vi "Dashboard Main.vi"() -> ()   [LabVIEW 2017]
uses:
  <vilib>/event_ctls.llb/eventvkey.ctl
  <vilib>/Rock Robotics/WPI/Dashboard/WPI_DashboardLogging Global.vi
  <vilib>/Utility/miscctls.llb/LVRowAndColumnTypeDef.ctl
  <vilib>/Rock Robotics/Network Tables/NT Write Boolean.vi
  <vilib>/Rock Robotics/Network Tables/NT Read Numeric Array.vi
panel:
  out "error out":errorcluster
  out "error out 2":errorcluster
  in  "Camera Settings Right":T1={"Frame Rate"=30, "Compression"=30, "Size"=1, "DB Camera Config"=FALSE} {"Frame Rate" scale=1.0..30.0; "Compression" scale=100.0..-1.0; "Size" items=["640x480", "320x240", "160x120"]}
  in  "Camera Name Right":string(combo)="No Camera Selection"
  out "Camera Info":cluster{"Mbps LED":bool, "Mbps":dbl, "fps":dbl} {"fps" format="%#.1g"; "Mbps" format="%#.1g"}
  in  "Camera Settings":T1={"Frame Rate"=30, "Compression"=30, "Size"=1, "DB Camera Config"=FALSE} {"Frame Rate" scale=1.0..30.0; "Compression" scale=100.0..-1.0; "Size" items=["640x480", "320x240", "160x120"]}
  in  "TCP":refnum<k5>
  in  "Rec Mode":enum32{"Stop", "Record", "Playback"}(radio)
  out "Robot IP":string
  out "Image Message":string="Timeout in Camera Communications"
  in  "Dashboard Tab":T2(tab)
  in  "Select Auto":string(combo)="Select Autonomous ..."
  out "NT Connection":bool
  out "MotorChart R":cluster{"Numeric":dbl, "Numeric":dbl}(graph)
  out "MotorChart L":cluster{"Numeric":dbl, "Numeric":dbl}(graph)
  out "MotorSliders R":cluster{"MotorSlide1":dbl, "MotorSlide2":dbl} {"MotorSlide2" scale=-1.0..1.0 scale format="%#_2e"; "MotorSlide1" scale=-1.0..1.0 scale format="%#_2e"}
  out "MotorSliders L":cluster{"MotorSlide1":dbl, "MotorSlide2":dbl} {"MotorSlide2" scale=-1.0..1.0 scale format="%#_2e"; "MotorSlide1" scale=-1.0..1.0 scale format="%#_2e"}
  out "JS1 Z":dbl(slide) scale=-1.0..1.0 scale format="%#_2e"
  out "JS1 Graph":cluster{"X":dbl, "Y":dbl}[](graph)
  out "JS1 Buttons":T3
  out "JS2 Z":dbl(slide) scale=-1.0..1.0 scale format="%#_2e"
  out "JS2 Graph":cluster{"X":dbl, "Y":dbl}[](graph)
  out "JS2 Buttons":T3
  out "Mode":T4(ring)=enum."Auto Disabled"
  out "Gear State":string="Waiting...."
  in  "Mode 2":bool
  out "Camera Image Right":T5(plugin-control)
  in  "DB/String 9":string
  in  "DB/String 8":string
  in  "DB/String 7":string
  in  "DB/String 6":string
  in  "DB/String 5":string
  in  "DB/String 4":string
  in  "DB/String 3":string
  in  "DB/String 2":string
  in  "DB/String 1":string
  in  "DB/String 0":string
  in  "DB/Slider 0":dbl(slide) scale=0.0..5.0
  in  "DB/Slider 1":dbl(slide) scale=0.0..5.0
  in  "DB/Slider 2":dbl(slide) scale=0.0..5.0
  in  "DB/Slider 3":dbl(slide) scale=0.0..5.0
  out "DB/LED 3":bool
  out "DB/LED 2":bool
  out "DB/LED 1":bool
  out "DB/LED 0":bool
  in  "DB/Button 3":bool
  in  "DB/Button 2":bool
  in  "DB/Button 1":bool
  in  "DB/Button 0":bool caption="New Name"
  in  "Test Slider":dbl(slide) scale=0.0..100.0 scale format="%#_3g"
  in  "On/Off":bool caption="Solenoid"
  in  "Test Name":u16(ring) items=["Select the test to run..."]
  in  "Test Tree":string(tree)
  in  "Motor":cluster{"Value":dbl, "Enable":bool} {"Value" scale=-1.0..1.0 scale format="%#_3g"}
  out "Progress":T6 {"Test Progress" scale=0.0..100.0}
  in  "Rev/Fwd":cluster{"Forward":bool, "Reverse":bool}
  in  "Test Ring":u16(ring) items=["Monochrome", "Color"]
  out "Cmd Status":string
  in  "Execute Command":bool
  in  "Command Params":string[][](table)
  in  "Command Selection":i32(listbox)
  in  "CheckList":i32(listbox)
  out "Tree":string(tree)
  in  "Max Speed":dbl=1.0 format="%#_13g"
  in  "Foreward Sensitivity":dbl=1.0 format="%#_13g"
  in  "Turning Sensitivity":dbl=0.4 format="%#_13g"
  in  "High Gear Turning Multiplier":dbl=0.65 format="%#_13g"
  in  "High Gear":bool=TRUE
  in  "Direction Toggle":bool=TRUE
  in  "Autoshift":bool=TRUE
  in  "Save":bool
  in  "Load":bool
  in  "Profile Name":string="Profile1"
  out "Camera Image":T5(plugin-control)
  out "Background":bool
  in  "Camera Name":string(combo)="No Camera Selection"
  # "HW"
  # "HW"
  # "Joysticks"
  # "Drive Motors"
  # "Front"
  # "Right"
  # "Left"
  # "Back"
  # "This tab is a great place for autonomous settings and robot-specific values.\nPlace controls and indicators inside this tab and match name to\nDashboard Variables on robot. You can also delete this comment."
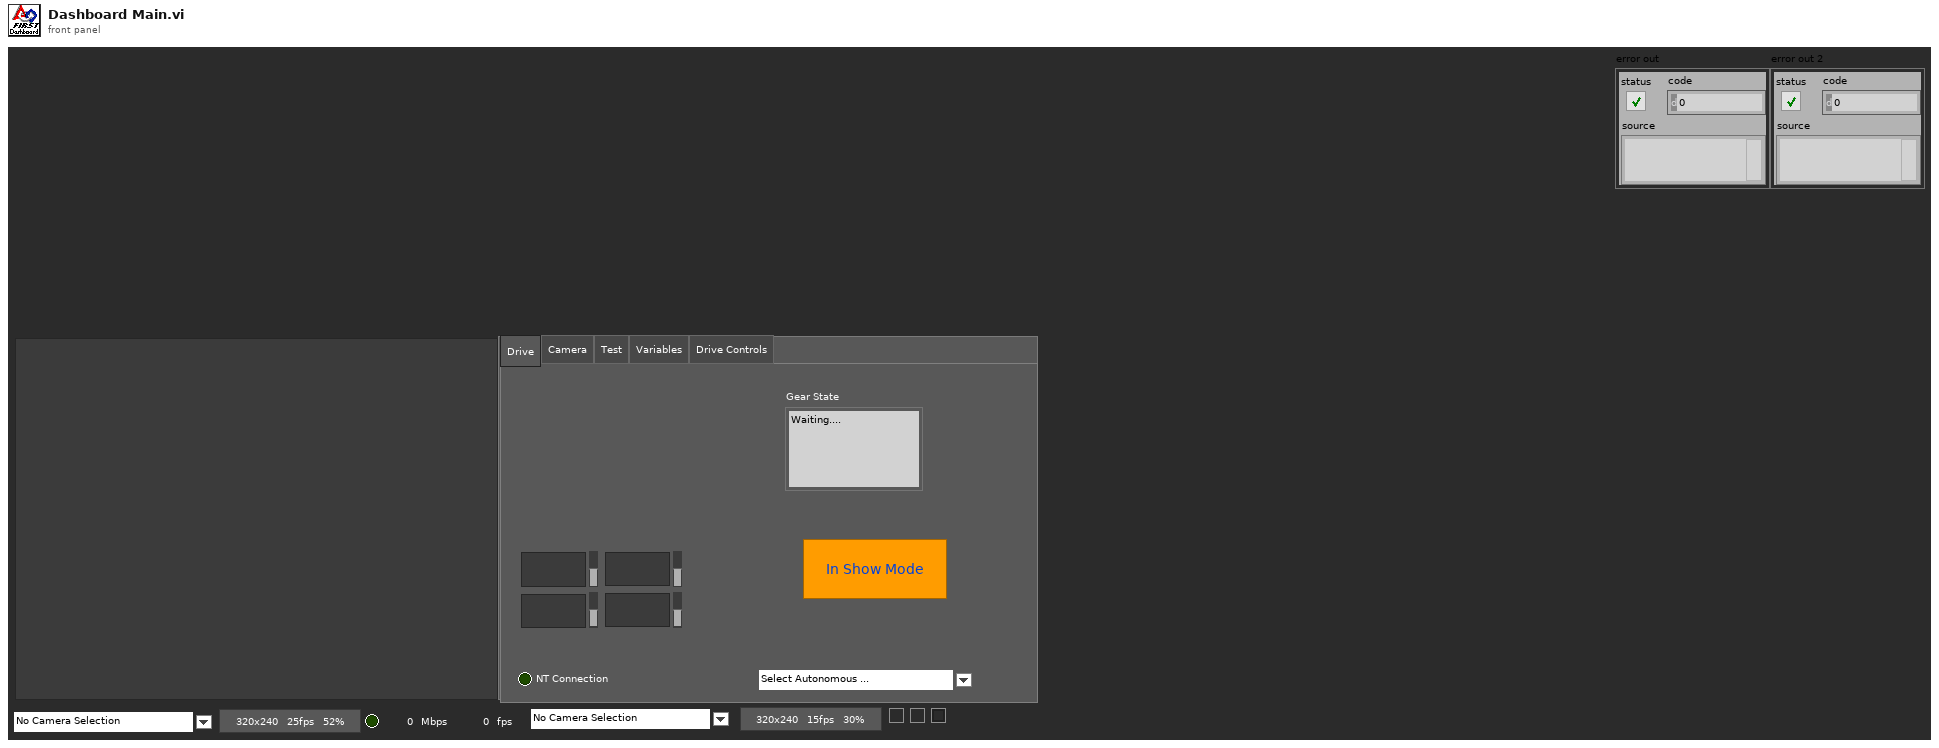
[diagram p1: front panel]
types:
  T1 = cluster{"Frame Rate":i32, "Compression":i32, "Size":u16, "DB Camera Config":bool}
  T2 = enum32{"Drive", "Camera", "Basic", "Custom", "Test", "Commands", "Checklist", "Variables", "Drive Controls"}
  T3 = cluster{bool, bool, bool, bool, bool, bool, bool, bool, bool, bool, bool, bool}
  T4 = enum8{"Tele-Op Disabled", "Tele-Op Enabled", "Auto Disabled", "Auto Enabled", "Test Disabled", "Test Enabled", "Disconnected", "No Code", "E-Stop"}
  T5 = typedef "IMAQ Image.ctl" = refnum<image>
  T6 = cluster{"Test Progress":u8, "Test Progress Text":string}
  T7 = typedef "Image Type" = u32
  T8 = cluster{"IDs":cluster{"RPC field ID":u16, "Unique ID":u16}, "String":string}
  T9 = enum32{"Drive", "Camera", "Basic", "Custom", "Test", "Commands", "Checklist", "Variables"}
  T10 = enum32{"Drive", "Basic", "Custom", "Test", "Checklist", "Variables"}
  T11 = cluster{"Error Strings":string, "Disable Counts":cluster{u16, u16}, "Rail Faults":cluster{u16, u16, u16}, "Robot IP":string, "DB Mode":u8, "Event Info":cluster{"Name":string, "Type":u8, "Number":u16, "Replay":u8}}
  T12 = cluster{"Storage":cluster{"Disk Free":u64, "RAM Block":u32, "RAM free":u32}, "CPU Utilization":cluster{"CPU % ISR":sgl, "CPU % Time Crit":sgl, "CPU % Timed Str":sgl, "CPU % High":sgl, "CPU % Above":sgl, "CPU % Normal":sgl, "CPU % Low":sgl}, "CAN":cluster{"% Bus Utilization":sgl, "Bus Off Cnt":u32, "TX_FIFO Full Cnt":u32, "Receive Error Cnt":u8, "Transmit Error Cnt":u8}, "HID":cluster{"HID Outputs":u32, "Rumble Low":u16, "Rumble High":u16}[]}
  T13 = cluster{"Status bits":cluster{"Test Mode":bool, "Autonomous":bool, "Enabled":bool, "Code Start":bool, "Brownout":bool, "Reserved 2":bool, "Reserved 3":bool, "E-Stop":bool}, "Code Trace":cluster{"Disabled":bool, "TeleOp":bool, "Auto":bool, "Test":bool}, "Controller Type":enum16{"unknown", "cRIO", "roboRio"}, "Code?":enum16{"unknown", "noCode", "code"}, "Battery V":dbl}
  T14 = cluster{"Control Bits":cluster{"TestMode":bool, "Autonomous":bool, "Enabled":bool, "FMS Present":bool, bool, bool, bool, "E-Stop":bool}, "Team Station ":u8, "Countdown":sgl, "Joystick Values":cluster{"Axes":dbl[], "Buttons":bool[], "POVs":i16[]}[]}
  T15 = cluster{"Axes":dbl[], "Buttons":bool[], "POVs":i16[]}[]
  T16 = cluster{"Axes":dbl[], "Buttons":bool[], "POVs":i16[]}
  T17 = cluster{"Buttons[0]":bool, "Buttons[1]":bool, "Buttons[2]":bool, "Buttons[3]":bool, "Buttons[4]":bool, "Buttons[5]":bool, "Buttons[6]":bool, "Buttons[7]":bool, "Buttons[8]":bool, "Buttons[9]":bool, "Buttons[10]":bool, "Buttons[11]":bool}
  T18 = cluster{"High Gear Turning Multiplier":refnum<vi>, "Turning Sensitivity":refnum<vi>, "Foreward Sensitivity":refnum<vi>, "Max Speed":refnum<vi>, "Autoshift":refnum<vi>, "High Gear":refnum<vi>, "Direction Toggle":refnum<vi>, "Profile Name":refnum<vi>}
  T19 = cluster{"Camera Image":refnum<vi>, "Dashboard Tab":refnum<vi>, "Background":refnum<vi>, "Rec Mode":refnum<vi>, "Test Slider":refnum<vi>, "On/Off ":refnum<vi>, "Test Ring":refnum<vi>, "Rev/Fwd":refnum<vi>, "Test Name":refnum<vi>, "Motor":refnum<vi>, "Progress":refnum<vi>, "CheckList":refnum<vi>, "Tree":refnum<vi>, "Test Tree":refnum<vi>, "Command Params":refnum<vi>, "Command Selection":refnum<vi>, "Execute Command":refnum<vi>, "Cmd Status":refnum<vi>, "Camera Settings":refnum<vi>, "Camera Name":refnum<vi>, "Camera Info":refnum<vi>, "Camera Settings Right":refnum<vi>, "Camera Name Right":refnum<vi>, "Camera Image Right":refnum<vi>}
  T20 = cluster{"Operation":enum16{"Update", "Clear"}, "Color Box":u32}[]
  T21 = typedef "eventvkey.ctl" = enum16{"ASCII", "Enter", "Return", "Shift", "Ctrl", "Alt", "Cmd", "Opt", "Caps", "NumLock", "Clear", "Break", "Up", "Down", "Left", "Right", "Insert", "Delete", "Home", "End", "PageUp", "PageDown", "Escape", "Help", "Pause", "ScrollLock", "F1", "F2", "F3", "F4", "F5", "F6", "F7", "F8", "F9", "F10", "F11", "F12", "F13", "F14", "F15", "F16", "F17", "F18", "F19", "F20", "F21", "F22", "F23", "F24", "Play", "VolumeUp", "VolumeDown", "Mute", "Two Byte Char"}
  T22 = cluster{"Image Size":bool, "Image Type":bool, "Pixel Value":bool, "ROI Information":bool, "Zoom Factor":bool}
  T23 = cluster{"Operation":enum16{"Update", "Clear"}, "Color Box":u32}
  T24 = typedef "LVRowAndColumnTypeDef.ctl" = cluster{"Row":i32, "Column":i32}
  T25 = cluster{"Shift":bool, "Ctrl":bool, "Alt":bool, "Cmd":bool, "Opt":bool}
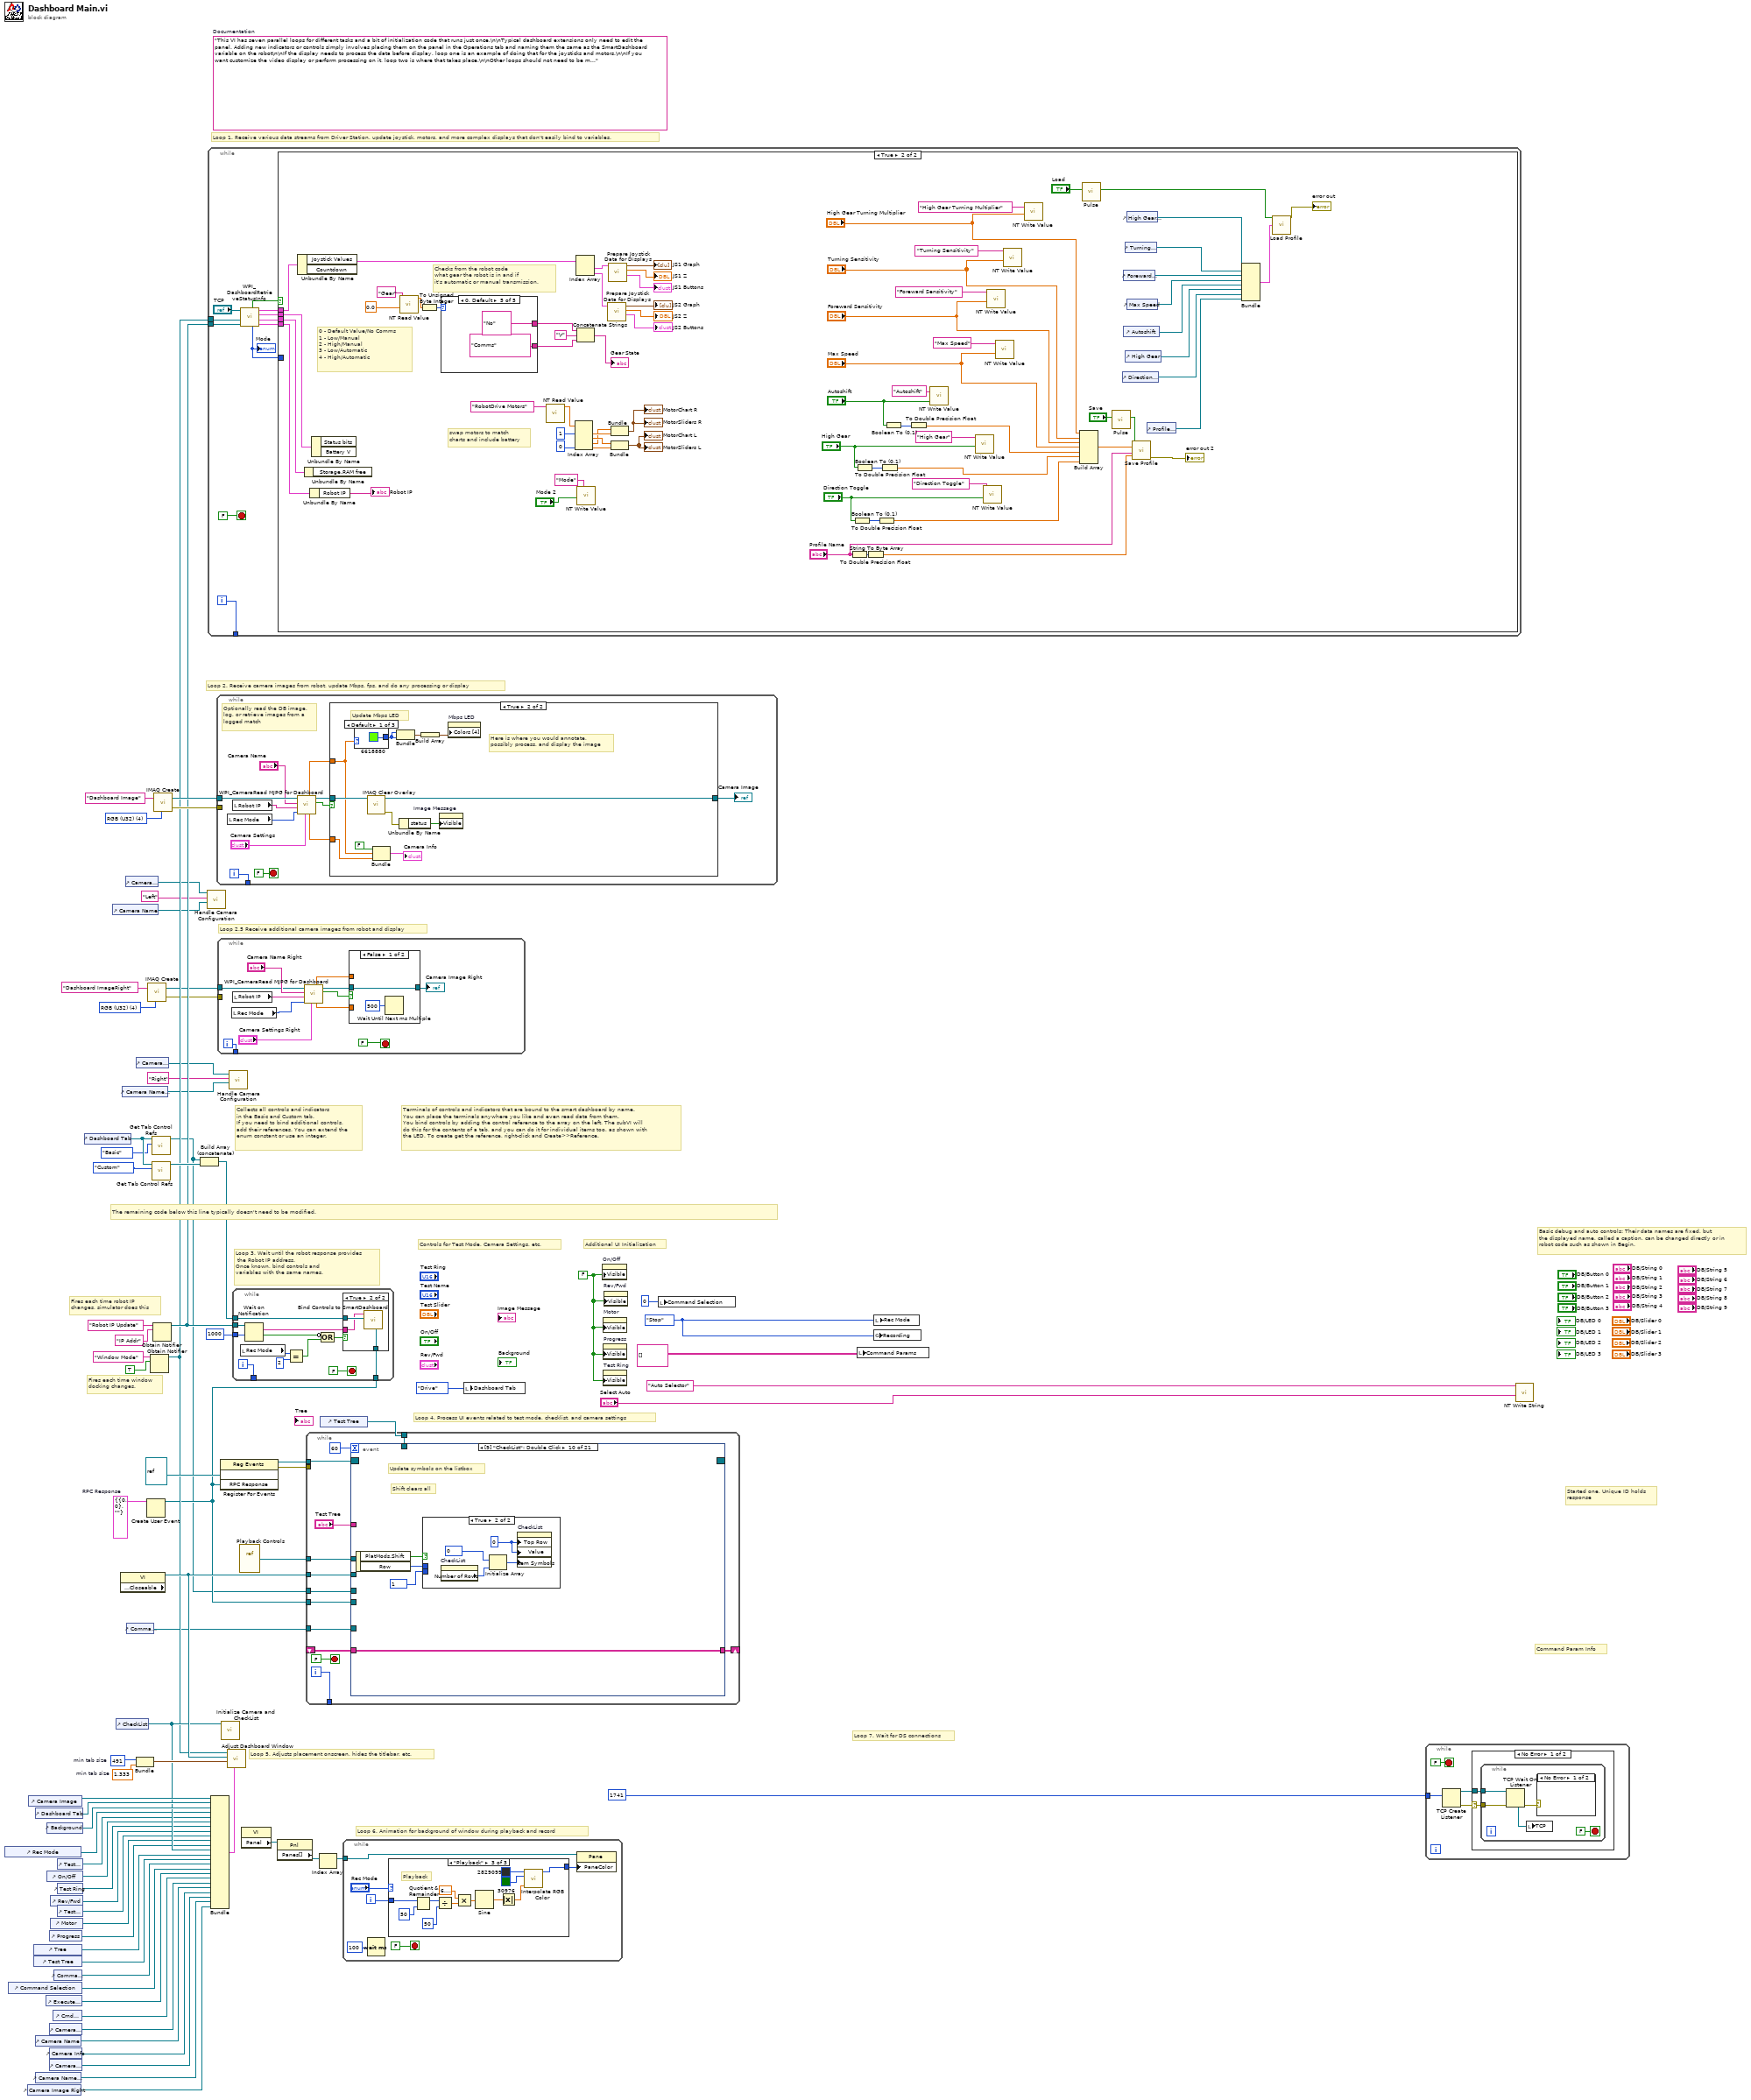
[diagram p0: block diagram]
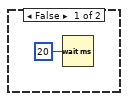
[diagram p3: hidden frame]
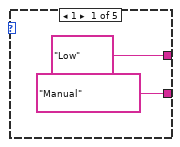
[diagram p4: hidden frame]
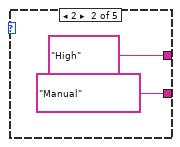
[diagram p5: hidden frame]
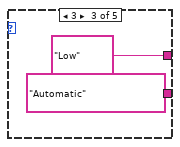
[diagram p6: hidden frame]
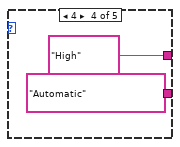
[diagram p7: hidden frame]
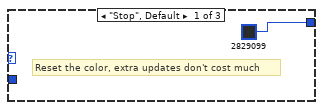
[diagram p8: hidden frame]
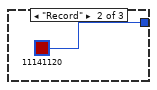
[diagram p9: hidden frame]
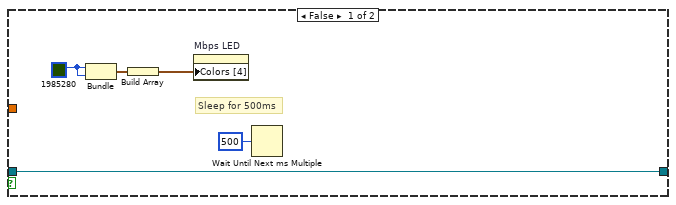
[diagram p11: hidden frame]
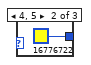
[diagram p12: hidden frame]
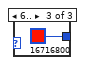
[diagram p13: hidden frame]
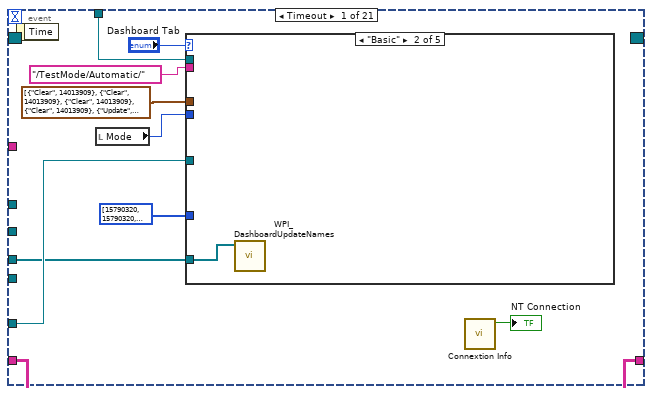
[diagram p14: hidden frame]
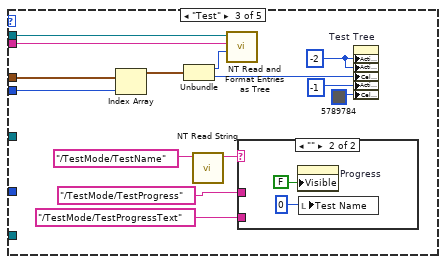
[diagram p16: hidden frame]
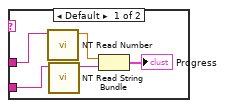
[diagram p17: hidden frame]
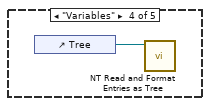
[diagram p18: hidden frame]
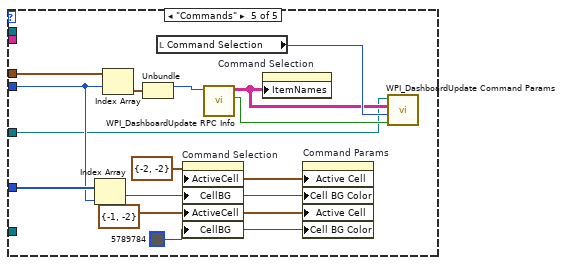
[diagram p19: hidden frame]
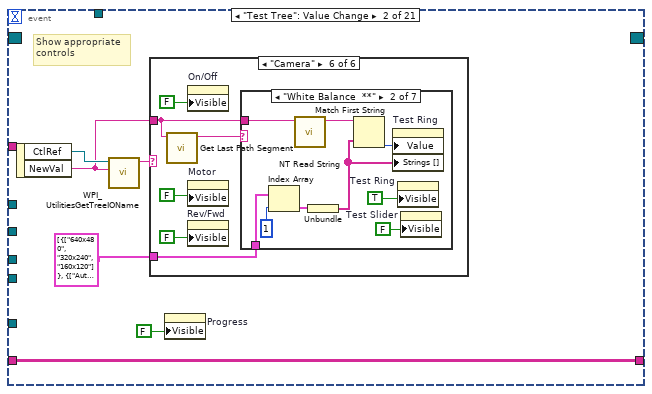
[diagram p20: hidden frame]
diagram:
  w10 = T7 4 items=["Grayscale (U8)", "Grayscale (I16)", "Grayscale (SGL)", "Complex (CSG)", "RGB (U32)", "HSL (U32)", "RGB (U64)"] ("Image Type")
  w26 = T8 {"IDs"={"RPC field ID"=0, "Unique ID"=0}, "String"=""}  # RPC Response
  w51 = 491  # min tab size
  w50 = 1.333  # min tab size
  w58 = enum32{"Stop", "Record", "Playback"}."Stop" ("Rec Mode")
  w33 = FALSE ("Visible")
  (unwired) "This VI has seven parallel loops for different tasks and a bit of initialization code that runs just once.\n\nTypical dashboard extensions only need to edit the panel. Adding new indicators or controls simply involves placing them on the panel in the Operations tab and naming them the same as the SmartDashboard variable on the robot\n\nIf the display needs to process the data before display, loop one is an example of doing that for the joysticks and motors.\n\nIf you want customize the video display or perform processing on it, loop two is where that takes place.\n\nOther loops should not need to be modified. They are pretty standard, and document the task they perform."  # Documentation
  w75 = T7 4 items=["Grayscale (U8)", "Grayscale (I16)", "Grayscale (SGL)", "Complex (CSG)", "RGB (U32)", "HSL (U32)", "RGB (U64)"] ("Image Type")
  # "Loop 2.5 Receive additional camera images from robot and display"
  # "Command Param Info"
  # "Started one, Unique ID holds\nresponse"
  # "Loop 7. Wait for DS connections"
  # "Basic debug and auto controls: Their data names are fixed, but\nthe displayed name, called a caption, can be changed directly or in\nrobot code such as shown in Begin."
  # "Controls for Test Mode, Camera Settings, etc."
  # "Additional UI Initialization"
  # "Loop 6. Animation for background of window during playback and record"
  # "Fires each time robot IP\nchanges, simulator does this"
  # "Fires each time window\ndocking changes."
  # "Collects all controls and indicators\nin the Basic and Custom tab.\nIf you need to bind additional controls,\nadd their references. You can extend the\nenum constant or use an integer."
  # "The remaining code below this line typically doesn't need to be modified."
  # "Loop 4. Process UI events related to test mode, checklist, and camera settings"
  # "Terminals of controls and indicators that are bound to the smart dashboard by name.\nYou can place the terminals anywhere you like and even read data from them.\nYou bind controls by adding the control reference to the array on the left. The subVI will\ndo this for the contents of a tab, and you can do it for individual items too, as shown with\nthe LED. To create get the reference, right-click and Create>>Reference."
  # "Loop 3. Wait until the robot response provides\n the Robot IP address.\nOnce known, bind controls and\nvariables with the same names."
  # "Loop 5. Adjusts placement onscreen, hides the titlebar, etc."
  # "Loop 1. Receive various data streams from Driver Station, update joystick, motors, and more complex displays that don't easily bind to variables."
  # "Loop 2. Receive camera images from robot, update Mbps, fps, and do any processing or display"
  n1 = control-ref of="Rec Mode"() -> (w39:refnum<vi>)
  n2 = control-ref of="Command Selection"() -> (w25:refnum<vi>)
  n3 = control-ref of="Camera Image Right"() -> (w1:refnum<vi>)
  n4 = control-ref of="Camera Image"() -> (w53:refnum<vi>)
  n5 = control-ref of="Tree"() -> (w43:refnum<vi>)
  n6 = control-ref of="Test Tree"() -> (w42:refnum<vi>)
  n7 = control-ref of="Dashboard Tab"() -> (w52:refnum<vi>)
  n8 = control-ref of="Camera Name"() -> (w16:refnum<vi>)
  n9 = control-ref of="Camera Name Right"() -> (w2:refnum<vi>)
  n10 = control-ref of="Execute Command"() -> (w27:refnum<vi>)
  n11 = control-ref of="Background"() -> (w48:refnum<vi>)
  n12 = control-ref of="On/Off"() -> (w37:refnum<vi>)
  n13 = control-ref of="Progress"() -> (w34:refnum<vi>)
  n14 = control-ref of="Camera Settings"() -> (w17:refnum<vi>)
  n15 = control-ref of="Camera Info"() -> (w15:refnum<vi>)
  n16 = control-ref of="Camera Settings Right"() -> (w3:refnum<vi>)
  n17 = control-ref of="Rev/Fwd"() -> (w35:refnum<vi>)
  n18 = control-ref of="Motor"() -> (w40:refnum<vi>)
  n19 = control-ref of="Cmd Status"() -> (w21:refnum<vi>)
  n20 = control-ref of="Command Params"() -> (w28:refnum<vi>)
  n21 = control-ref of="Test Slider"() -> (w38:refnum<vi>)
  n22 = control-ref of="Test Ring"() -> (w36:refnum<vi>)
  n23 = control-ref of="Test Name"() -> (w41:refnum<vi>)
  n24 = control-ref of="Dashboard Tab"() -> (w56:refnum<vi>)
  n25 = control-ref of="Camera Name"() -> (w18:refnum<vi>)
  n26 = control-ref of="CheckList"() -> (w44:refnum<vi>)
  n27 = property class="VI" props=["Front Panel.Closeable"]() -> (reference out=w57:refnum<vi>)  [unwired: 2 in, 2 out]
  n28 = control-ref of="Camera Name Right"() -> (w6:refnum<vi>)
  n29 = control-ref of="Camera Settings"() -> (w19:refnum<vi>)
  n30 = control-ref of="Command Params"() -> (w20:refnum<vi>)
  n31 = control-ref of="Camera Settings Right"() -> (w7:refnum<vi>)
  n32 = Bundle("min tab size"=w51, "min tab size"=w50) -> (w49:cluster{"min tab size":i32, "min tab size":dbl})  [unwired: 1 in]
  n33 = Create User Event(user event datatype=w26) -> (user event=w22:refnum<user-event>)  [unwired: 1 in, 1 out]
  n34 = call "IMAQ Create"("Image Name"="Dashboard ImageRight", "Image Type"=w10) -> ("New Image"=w9:T5, "error out"=w8:errorcluster)  [unwired: 2 in, 1 out]
  n35 = Obtain Notifier(name (unnamed)="Window Mode", notification data type=TRUE) -> (notifier out=w31:refnum<notifier>)  [unwired: 2 in, 2 out]
  n36 = call <vilib>:"Get Tab Control Refs.vi"("Page Index"=T10."Basic" ("Dashboard Tab"), "TabControl in"=w56) -> ("ControlsOnPage"=w14:refnum<vi>[])  [unwired: 9 in]
  n37 = call <vilib>:"Get Tab Control Refs.vi"("Page Index"=T10."Custom" ("Dashboard Tab"), "TabControl in"=w56) -> ("ControlsOnPage"=w55:refnum<vi>[])  [unwired: 9 in]
  n38 = Obtain Notifier(name (unnamed)="Robot IP Update", notification data type="IP Addr" ("name (unnamed)")) -> (notifier out=w32:refnum<notifier>)  [unwired: 2 in, 2 out]
  n39 = call "IMAQ Create"("Image Name"="Dashboard Image", "Image Type"=w75) -> ("New Image"=w73:T5, "error out"=w72:errorcluster)  [unwired: 2 in, 1 out]
  n40 = Build Array (concatenate)(w14, w55) -> (w54:refnum<vi>[])
  n41 = call "Handle Camera Configuration.vi"("CameraNameRef"=w18, "Camera File Name"="Left", "ClusterRef"=w19) -> ()  [unwired: 9 in]
  n42 = while {
    tunnel: [w85] -> _
    tunnel: w32 -> [w79]
    tunnel: w31 -> [w76]
    i -> [w85]
    stop <- FALSE stop-if-true
    n43 = call <vilib>:"WPI_DashboardRetrieveStatusInfo.vi"("Binding Refnum"=w79, "Window Mode Notifier"=w76, "TCP Cnx"="TCP") -> ("Power and Errors"=w80:T11, "Robot Metrics"=w83:T12, "Status Info"=w84:T13, "Control Info"=w81:T14, "Robot Mode"=w78:T4, "Process?"=w82:bool)  [unwired: 3 in]
    "Mode" <- w78
    n44 = case shown="True" w82 {
      tunnel: w84 -> [_ w160]
      tunnel: w83 -> [_ w159]
      tunnel: w81 -> [_ w158]
      tunnel: w80 -> [_ w157]
      tunnel: w78 -> [_ _]
      frame False {
        n45 = Wait (ms)(milliseconds to wait=u32 20) -> ()  [unwired: 1 out]
      }
      frame True {
        # "Checks from the robot code\nwhat gear the robot is in and if\nit's automatic or manual transmission."
        # "0 - Default Value/No Comms\n1 - Low/Manual\n2 - High/Manual\n3 - Low/Automatic\n4 - High/Automatic"
        # "swap motors to match\ncharts and include battery"
        n46 = Unbundle By Name(w158) -> ("Joystick Values"=w148:T15)  [unwired: 1 out]
        n47 = Unbundle By Name(w159) -> ()  [unwired: 1 out]
        n48 = Unbundle By Name(w157) -> ("Robot IP"=→"Robot IP":string)
        n49 = Unbundle By Name(w160) -> ()  [unwired: 2 out]
        n50 = call-poly <vilib>:"NT Read Value.vi"("Default Value"=0.0, "Name"="Gear") -> ("Numeric"=w129:dbl)  [unwired: 8 in, 1 out]
        n51 = To Unsigned Byte Integer(number=w129) -> (unsigned 8bit integer=w130:u8)
        n52 = case shown="0, Default" w130 {
          tunnel: ["Low" "High" "Low" "High" "No"] -> w134
          tunnel: ["Manual" "Manual" "Automatic" "Automatic" "Comms"] -> w132
          frame 1 {
          }
          frame 2 {
          }
          frame 3 {
          }
          frame 4 {
          }
          frame 0, Default {
          }
        }
        n53 = call-poly <vilib>:"NT Read Value.vi"("Name"="RobotDrive Motors") -> ("Numeric Array"=w138:dbl[])  [unwired: 9 in, 1 out]
        n54 = Index Array(array=w138, index #1=1, index #4=0) -> (element #1=w152:dbl, element #2=w153:dbl, element #3=w151:dbl, element #4=w156:dbl)  [unwired: 2 in]
        n55 = Index Array(array=w148) -> (element #1=w147:T16, element #2=w143:T16)  [unwired: 2 in]
        n56 = Concatenate Strings(w134, "\r", w132) -> (→"Gear State":string)
        n57 = call-poly <vilib>:"NT Write Value.vi"("Boolean"="Mode 2", "Name"="Mode") -> ()  [unwired: 9 in, 1 out]
        n58 = call "Prepare Joystick Data for Displays.vi"("Joystick Values"=w143) -> ("Buttons"=→"JS2 Buttons":T17, "Z Axis"=→"JS2 Z":dbl, "Cartesian Data"=→"JS2 Graph":cluster{"X axis":dbl, "X axis":dbl}[])  [unwired: 8 in]
        n59 = call "Prepare Joystick Data for Displays.vi"("Joystick Values"=w147) -> ("Buttons"=→"JS1 Buttons":T17, "Z Axis"=→"JS1 Z":dbl, "Cartesian Data"=→"JS1 Graph":cluster{"X axis":dbl, "X axis":dbl}[])  [unwired: 8 in]
        n60 = Bundle("Numeric"=w151, "Numeric"=w152) -> (→"MotorChart R" →"MotorSliders R":cluster{"Numeric":dbl, "Numeric":dbl})  [unwired: 1 in]
        n61 = Bundle("Numeric"=w153, "Numeric"=w156) -> (→"MotorChart L" →"MotorSliders L":cluster{"Numeric":dbl, "Numeric":dbl})  [unwired: 1 in]
        n62 = String To Byte Array(string="Profile Name") -> (unsigned byte array=w109:u8[])
        n63 = Boolean To (0,1)(Boolean="Direction Toggle") -> (0, 1=w106:i16)
        n64 = Boolean To (0,1)(Boolean="High Gear") -> (0, 1=w104:i16)
        n65 = To Double Precision Float(number=w109) -> (double precision float=w111:dbl[])
        n66 = To Double Precision Float(number=w106) -> (double precision float=w107:dbl)
        n67 = To Double Precision Float(number=w104) -> (double precision float=w105:dbl)
        n68 = Boolean To (0,1)(Boolean="Autoshift") -> (0, 1=w102:i16)
        n69 = To Double Precision Float(number=w102) -> (double precision float=w103:dbl)
        n70 = call-poly <vilib>:"NT Write Value.vi"("Boolean"="Autoshift", "Name"="Autoshift") -> ()  [unwired: 9 in, 1 out]
        n71 = call-poly <vilib>:"NT Write Value.vi"("Boolean"="High Gear", "Name"="High Gear") -> ()  [unwired: 9 in, 1 out]
        n72 = call-poly <vilib>:"NT Write Value.vi"("Boolean"="Direction Toggle", "Name"="Direction Toggle") -> ()  [unwired: 9 in, 1 out]
        n73 = call-poly <vilib>:"NT Write Value.vi"("Numeric"="Foreward Sensitivity", "Name"="Foreward Sensitivity") -> ()  [unwired: 9 in, 1 out]
        n74 = call-poly <vilib>:"NT Write Value.vi"("Numeric"="Max Speed", "Name"="Max Speed") -> ()  [unwired: 9 in, 1 out]
        n75 = call-poly <vilib>:"NT Write Value.vi"("Numeric"="Turning Sensitivity", "Name"="Turning Sensitivity") -> ()  [unwired: 9 in, 1 out]
        n76 = call-poly <vilib>:"NT Write Value.vi"("Numeric"="High Gear Turning Multiplier", "Name"="High Gear Turning Multiplier") -> ()  [unwired: 9 in, 1 out]
        n77 = Build Array("High Gear Turning Multiplier", "Turning Sensitivity", "Foreward Sensitivity", "Max Speed", w103, w105, w107) -> (w110:dbl[])
        n78 = call "Pulse.vi"("Input"="Load") -> ("Output"=w98:bool)  [unwired: 10 in]
        n79 = call "Pulse.vi"("Input"="Save") -> ("Output"=w101:bool)  [unwired: 10 in]
        n80 = control-ref of="Direction Toggle"() -> (w90:refnum<vi>)
        n81 = control-ref of="Autoshift"() -> (w92:refnum<vi>)
        n82 = control-ref of="Foreward Sensitivity"() -> (w94:refnum<vi>)
        n83 = control-ref of="High Gear"() -> (w91:refnum<vi>)
        n84 = control-ref of="Turning Sensitivity"() -> (w95:refnum<vi>)
        n85 = control-ref of="High Gear Turning Multiplier"() -> (w96:refnum<vi>)
        n86 = control-ref of="Max Speed"() -> (w93:refnum<vi>)
        n87 = call "Save Profile.vi"("Array 2"=w111, "Profile Name"="Profile Name", "Array"=w110, "Output"=w101) -> ("error out"=→"error out 2":errorcluster)  [unwired: 7 in]
        n88 = control-ref of="Profile Name"() -> (w89:refnum<vi>)
        n89 = Bundle("High Gear Turning Multiplier"=w96, "Turning Sensitivity"=w95, "Foreward Sensitivity"=w94, "Max Speed"=w93, "Autoshift"=w92, "High Gear"=w91, "Direction Toggle"=w90, "Profile Name"=w89) -> (w88:T18)  [unwired: 1 in]
        n90 = call "Load Profile.vi"("Output"=w98, "output cluster"=w88) -> ("error out"=→"error out":errorcluster)  [unwired: 13 in]
      }
    }
  }
  n91 = Bundle("Camera Image"=w53, "Dashboard Tab"=w52, "Background"=w48, "Rec Mode"=w39, "Test Slider"=w38, "On/Off"=w37, "Test Ring"=w36, "Rev/Fwd"=w35, "Test Name"=w41, "Motor"=w40, "Progress"=w34, "CheckList"=w44, "Tree"=w43, "Test Tree"=w42, "Command Params"=w28, "Command Selection"=w25, "Execute Command"=w27, "Cmd Status"=w21, "Camera Settings"=w17, "Camera Name"=w16, "Camera Info"=w15, "Camera Settings Right"=w3, "Camera Name Right"=w2, "Camera Image Right"=w1) -> (w45:T19)  [unwired: 1 in]
  n92 = while {
    tunnel: w73 -> [w180]
    tunnel: w72 -> [_]
    tunnel: [w181] -> _
    i -> [w181]
    stop <- FALSE stop-if-true
    # "Optionally read the DB image,\nlog, or retrieve images from a\nlogged match"
    n93 = local read "Rec Mode"() -> (w176:enum32{"Stop", "Record", "Playback"})
    n94 = local read "Robot IP"() -> (w175:string)
    n95 = call <vilib>:"WPI_CameraRead MJPG for Dashboard.vi"("Camera Settings"="Camera Settings", "Rec Mode"=w176, "NT Connection"=w175, "Capture Info"="Camera Name", "Refnum in"=w180) -> ("Active"=w178:bool, "Refnum out"=w179:T5, "FPS"=w177:dbl, "Bandwidth (Mbps)"=w174:dbl)  [unwired: 3 in]
    n96 = case shown="True" w178 {
      tunnel: w179 -> [w183 w194]
      tunnel: w174 -> [_ w191]
      tunnel: w177 -> [_ w192]
      tunnel: [w183 w188] -> w171
      frame False {
        w185 = u32 1985280 ("Color Box")
        # "Sleep for 500ms"
        n97 = Bundle("Color Box"=w185, "Color Box"=w185) -> (w186:cluster{"Color Box":u32, "Color Box":u32})  [unwired: 1 out]
        n98 = Build Array(w186) -> (w184:cluster{"Color Box":u32, "Color Box":u32}[])
        n99 = property on="Mbps LED" class="Bool (strict)"("Colors [4]"=w184) -> ()  [unwired: 2 in, 2 out]
        n100 = Wait Until Next ms Multiple(millisecond multiple=u32 500) -> ()  [unwired: 1 out]
      }
      frame True {
        # "Here is where you would annotate,\npossibly process, and display the image"
        # "Update Mbps LED"
        n101 = case shown="Default" w191 {
          tunnel: [u32 6618880 ("Color Box") u32 16776722 ("Color Box") u32 16716800 ("Color Box")] -> w195
          frame Default {
          }
          frame 4, 5 {
          }
          frame 6.. {
          }
        }
        n102 = call "IMAQ Clear Overlay"("Image"=w194) -> ("error out"=w197:errorcluster, "Image Out"=w188:T5)  [unwired: 2 in, 7 out]
        n103 = Bundle(FALSE, "Bandwidth (Mbps)"=w191, "FPS"=w192) -> (→"Camera Info":cluster{bool, "Bandwidth (Mbps)":dbl, "FPS":dbl})  [unwired: 1 in]
        n104 = Bundle("Color Box"=w195, "Color Box"=w195) -> (w196:cluster{"Color Box":u32, "Color Box":u32})  [unwired: 1 out]
        n105 = Unbundle By Name(w197) -> ("status"=w198:bool)
        n106 = Build Array(w196) -> (w193:cluster{"Color Box":u32, "Color Box":u32}[])
        n107 = property on="Image Message" class="Str"("Visible"=w198) -> ()  [unwired: 2 in, 2 out]
        n108 = property on="Mbps LED" class="Bool (strict)"("Colors [4]"=w193) -> ()  [unwired: 2 in, 2 out]
      }
    }
    "Camera Image" <- w171
  }
  n109 = while {
    tunnel: w9 -> [w212]
    tunnel: w8 -> [_]
    tunnel: [w206] -> _
    i -> [w206]
    stop <- FALSE stop-if-true
    n110 = local read "Rec Mode"() -> (w210:enum32{"Stop", "Record", "Playback"})
    n111 = local read "Robot IP"() -> (w211:string)
    n112 = call <vilib>:"WPI_CameraRead MJPG for Dashboard.vi"("Camera Settings"="Camera Settings Right", "Rec Mode"=w210, "NT Connection"=w211, "Capture Info"="Camera Name Right", "Refnum in"=w212) -> ("Active"=w205:bool, "Refnum out"=w208:T5, "FPS"=w203:dbl, "Bandwidth (Mbps)"=w204:dbl)  [unwired: 3 in]
    n113 = case shown="False" w205 {
      tunnel: w208 -> [w214 w216]
      tunnel: w204 -> [_ _]
      tunnel: w203 -> [_ _]
      tunnel: [w214 w216] -> w202
      frame False {
        n114 = Wait Until Next ms Multiple(millisecond multiple=u32 500) -> ()  [unwired: 1 out]
      }
      frame True {
      }
    }
    "Camera Image Right" <- w202
  }
  n115 = register-events(refnum<vi> refnum, w22) -> (reference out=w62:refnum<event-registration>, error out=w61:errorcluster)  [unwired: 2 in]
  n116 = call "Initialize Camera and CheckList.vi"("ListBox in"=w44) -> ()  [unwired: 11 in]
  n117 = call "Adjust Dashboard Window.vi"("Sizing Refnums"=w45, "Size Constraints"=w49, "VI"=w57, "WIn Mode"=w31) -> ()  [unwired: 8 in]
  n118 = call "Handle Camera Configuration.vi"("CameraNameRef"=w6, "Camera File Name"="Right", "ClusterRef"=w7) -> ()  [unwired: 9 in]
  n119 = while {
    tunnel: w54 -> [w228]
    tunnel: w32 -> [w226]
    tunnel: [w224] -> _
    tunnel: u32 1000 ("milliseconds to wait") -> [w223]
    tunnel: w22 -> [w217]
    i -> [w224]
    stop <- FALSE stop-if-true
    n120 = local read "Rec Mode"() -> (w219:enum32{"Stop", "Record", "Playback"})
    n121 = Wait on Notification(notifier=w226, timeout in ms (-1)=w223) -> (notification=w225:string, timed out?=w221:bool)  [unwired: 2 in, 2 out]
    n122 = Equal?(x=w219, y=u16 2 ("Rec Mode")) -> (x = y?=w220:bool)
    n123 = Compound Arithmetic op=OR(invert w221, w220) -> (w222:bool)
    n124 = case shown="True" w222 {
      tunnel: w228 -> [_ w231]
      tunnel: w225 -> [_ w230]
      tunnel: w217 -> [_ w229]
      frame False {
      }
      frame True {
        n125 = call <vilib>:"Bind Controls to SmartDashboard.vi"("RPC ref"=w229, "Bound Control Refs"=w231, "Server IP Address"=w230) -> ()  [unwired: 9 in]
      }
    }
  }
  n126 = vi-ref "Playback Controls.vi"() -> (w63:refnum<vi>)
  n127 = property class="VI"() -> ("Panel"=w65:refnum<vi>)  [unwired: 2 in, 2 out]
  n128 = property class="Pnl"(reference=w65) -> ("Panes[]"=w66:refnum<vi>[])  [unwired: 1 in, 2 out]
  n129 = Index Array(array=w66) -> (element=w64:refnum<vi>)  [unwired: 1 in]
  n130 = control-ref of="Test Tree"() -> (w67:refnum<vi>)
  n131 = while {
    tunnel: [w241] -> _
    tunnel: w67 -> [w240]
    tunnel: w63 -> [w239]
    tunnel: w62 -> [w238]
    tunnel: w61 -> [_]
    tunnel: w57 -> [w237]
    tunnel: w22 -> [w236]
    tunnel: w20 -> [w235]
    shift-right: [w234] -> _
    shift-left: _ -> [w233]
    tunnel: w14 -> [w232]
    i -> [w241]
    stop <- FALSE stop-if-true
    n132 = event shown="[9] \"CheckList\": Double Click" {
      selector: w238 -> [_ _ _ _ _ _ _ _ _ _ _ _ _ _ _ _ _ _ _ _ _]
      dyn-events: [_ _ _ _ _ _ _ _ _ _ _ _ _ _ _ _ w497 _ _ _ _] -> _
      timeout: u32 60 ("milliseconds to wait") -> [_ _ _ _ _ _ _ _ _ _ _ _ _ _ _ _ _ _ _ _ _]
      tunnel: w240 -> [w253 _ _ _ _ _ _ _ _ _ _ _ _ _ _ _ _ _ _ _ _]
      tunnel: "Test Tree" -> [_ _ _ _ _ _ _ _ _ _ _ w464 w472 w474 w478 w486 _ _ _ _ _]
      tunnel: w239 -> [_ _ _ _ _ _ _ _ _ _ _ _ _ _ _ _ w499 _ w517 _ _]
      tunnel: w237 -> [_ _ _ _ _ _ _ _ _ _ _ _ _ _ _ _ w495 _ _ _ _]
      tunnel: w236 -> [_ _ _ _ _ _ _ _ _ _ _ _ _ _ _ _ w491 _ _ _ _]
      tunnel: w235 -> [w248 _ _ _ _ _ w415 _ _ _ _ _ _ _ _ _ _ _ _ _ _]
      tunnel: [w247 w292 w394 w399 w408 w412 w413 w422 w432 w439 w451 w463 w470 w473 w477 w485 w490 w512 w514 w518 w529] -> w234
      tunnel: w233 -> [w247 w292 w394 w399 w408 w412 w413 _ _ w439 w451 w463 w470 w473 w477 w485 w490 w512 w514 w518 w529]
      tunnel: w232 -> [w245 _ _ _ _ _ _ _ _ _ _ _ _ _ _ _ _ _ _ _ _]
      event Timeout {
        n133 = event-data() -> ()  [unwired: 1 in, 1 out]
        n134 = local read "Mode"() -> (w250:T4)
        n135 = case shown="\"Basic\"" "Dashboard Tab" {
          tunnel: w253 -> [_ _ w269 _ _]
          tunnel: "/TestMode/Automatic/" ("Name Pattern") -> [_ _ w268 _ _]
          tunnel: T20 [{"Operation"=enum."Clear", "Color Box"=14013909}, {"Operation"=enum."Clear", "Color Box"=14013909}, {"Operation"=enum."Clear", "Color Box"=14013909}, {"Operation"=enum."Clear", "Color Box"=14013909}, {"Operation"=enum."Update", "Color Box"=14013909}, {"Operation"=enum."Update", "Color Box"=16777215}, {"Operation"=enum."Clear", "Color Box"=14013909}, {"Operation"=enum."Clear", "Color Box"=14013909}, {"Operation"=enum."Clear", "Color Box"=14013909}] -> [_ _ w261 _ w285]
          tunnel: w250 -> [_ _ w260 _ w284]
          tunnel: u32[] [15790320, 15790320, 15790320, 15790320, 16777215, 16777215, 15790320, 15790320, 15790320] -> [_ _ _ _ w290]
          tunnel: w248 -> [_ _ _ _ w278]
          tunnel: w245 -> [_ w255 _ _ _]
          frame "Custom", Default {
          }
          frame "Basic" {
            n136 = call <vilib>:"WPI_DashboardUpdateNames.vi"("Controls on Tab"=w255) -> ()  [unwired: 11 in]
          }
          frame "Test" {
            w267 = -2 ("Active Item:Row Number")
            n137 = Index Array(array=w261, index=w260) -> (element=w262:T23)
            n138 = Unbundle(w262) -> ("Operation"=w263:enum16{"Update", "Clear"}, "Color Box"=w264:u32)
            n139 = call <vilib>:"NT Read String.vi"("Name"="/TestMode/TestName") -> ("String"=w258:string)  [unwired: 9 in, 1 out]
            n140 = call <vilib>:"NT Read and Format Entries as Tree.vi"("Operation"=w263, "Name Pattern"=w268, "Tree Refnum"=w269) -> ()  [unwired: 7 in, 2 out]
            n141 = case shown="\"\"" w258 {
              tunnel: "/TestMode/TestProgress" ("Name") -> [w271 _]
              tunnel: "/TestMode/TestProgressText" ("Name") -> [w270 _]
              frame Default {
                n142 = call <vilib>:"NT Read Number.vi"("Name"=w271) -> ("Numeric"=w272:dbl)  [unwired: 9 in, 1 out]
                n143 = call <vilib>:"NT Read String.vi"("Name"=w270) -> ("String"=w273:string)  [unwired: 9 in, 1 out]
                n144 = Bundle("Numeric"=w272, "String"=w273) -> (→"Progress":cluster{"Numeric":dbl, "String":string})  [unwired: 1 in]
              }
              frame "" {
                n145 = property on="Progress" class="Clust (strict)"("Visible"=FALSE) -> ()  [unwired: 2 in, 2 out]
                n146 = local write "Test Name"(u16 0) -> ()
              }
            }
            n147 = property on="Test Tree" class="Tree (strict)"("Active Item Row Number"=w267, "ActiveColNum"=w267, "CellBG"=w264, "Active Item Row Number"=-1 ("Active Item:Row Number"), "CellBG"=u32 5789784 ("Color Box")) -> ()  [unwired: 2 in, 2 out]
          }
          frame "Variables" {
            n148 = control-ref of="Tree"() -> (w277:refnum<vi>)
            n149 = call <vilib>:"NT Read and Format Entries as Tree.vi"("Tree Refnum"=w277) -> ()  [unwired: 9 in, 2 out]
          }
          frame "Commands" {
            w286 = u32 5789784 ("Color Box")
            w287 = T24 {"Row"=-1, "Column"=-2} ("Active Cell:Active Cell")
            w289 = T24 {"Row"=-2, "Column"=-2} ("Active Cell:Active Cell")
            n150 = Index Array(array=w290, index=w284) -> (element=w288:u32)
            n151 = Index Array(array=w285, index=w284) -> (element=w283:T23)
            n152 = Unbundle(w283) -> ("Operation"=w282:enum16{"Update", "Clear"})  [unwired: 1 out]
            n153 = local read "Command Selection"() -> (w281:i32)
            n154 = property on="Command Selection" class="MCListbox (strict)"("ActiveCell"=w289, "CellBG"=w288, "ActiveCell"=w287, "CellBG"=w286) -> ()  [unwired: 2 in, 2 out]
            n155 = call <vilib>:"WPI_DashboardUpdate RPC Info.vi"("Operation"=w282) -> ("update"=w280:bool, "commands"=w279:string[][])  [unwired: 9 in]
            n156 = property on="Command Selection" class="MCListbox (strict)"("ItemNames"=w279) -> ()  [unwired: 2 in, 2 out]
            n157 = property on="Command Params" class="Tbl (strict)"("Active Cell"=w289, "Cell BG Color"=w288, "Active Cell"=w287, "Cell BG Color"=w286) -> ()  [unwired: 2 in, 2 out]
            n158 = call <vilib>:"WPI_DashboardUpdate Command Params.vi"("Update"=w280, "NewVal"=w281, "Commands"=w279, "Param Tbl"=w278) -> ()  [unwired: 7 in, 1 out]
          }
        }
        n159 = call <vilib>:"Connextion Info.vi"() -> ("Connected"=→"NT Connection":bool)  [unwired: 10 in, 1 out]
      }
      event "Test Tree": Value Change {
        # "Show appropriate\ncontrols"
        n160 = event-data() -> ("CtlRef"=w295:refnum<vi>, "NewVal"=w293:string)  [unwired: 1 in]
        n161 = call <vilib>:"WPI_UtilitiesGetTreeIOName.vi"("NewVal"=w293, "TreeControl in"=w295) -> ("I/O Name"=w296:string)  [unwired: 9 in]
        n162 = case shown="\"Camera\"" w296 {
          selector: w296 -> [_ w303 _ w325 w334 _]
          tunnel: w293 -> [_ _ w322 w324 _ w341]
          tunnel: cluster{string[]}[] [{["640x480", "320x240", "160x120"]}, {["Auto", "Fixed indoor", "Fixed outdoor 1", "Fixed outdoor 2", "Fixed fluorescent 1", "Fixed fluorescent 2", "Hold current"]}, {["Auto", "Flicker-free 50 Hz", "Flicker-free 60 Hz", "Hold current"]}, {["None", "Prioritize frame rate", "Prioritize image quality"]}, {["Monochrome", "Color"]}] -> [_ _ _ _ _ w340]
          frame Default {
            w298 = FALSE ("Visible")
            w297 = FALSE ("Visible")
            n163 = property on="Motor" class="Clust (strict)"("Visible"=w297) -> ()  [unwired: 2 in, 2 out]
            n164 = property on="Test Ring" class="Ring (strict)"("Visible"=w297) -> ()  [unwired: 2 in, 2 out]
            n165 = property on="Rev/Fwd" class="Clust (strict)"("Visible"=w298) -> ()  [unwired: 2 in, 2 out]
            n166 = property on="On/Off" class="Bool (strict)"("Visible"=w298) -> ()  [unwired: 2 in, 2 out]
            n167 = property on="Test Slider" class="Slide (strict)"("Visible"=w298) -> ()  [unwired: 2 in, 2 out]
          }
          frame "Analog Out", "Motor", "PWM" {
            w304 = FALSE ("Visible")
            n168 = case shown="\"Analog Out\"" w303 {
              tunnel: [1.0 ("Value") -1.0 ("Value") 0.0 ("Value")] -> w302
              tunnel: [255.0 ("Value") 1.0 ("Value") 5.0 ("Value")] -> w301
              tunnel: [128.0 ("Value") 0.0 ("Value") 0.0 ("Value")] -> w300
              tunnel: [64.0 ("Value") 0.5 ("Value") 1.0 ("Value")] -> w299
              frame "PWM" {
              }
              frame "Motor", Default {
              }
              frame "Analog Out" {
              }
            }
            n169 = property on="Motor" class="Clust (strict)"("Visible"=TRUE) -> ()  [unwired: 2 in, 2 out]
            n170 = property on="Value" class="Slide (strict)"("Value"=w300, "Scale.Minimum"=w302, "Scale.Maximum"=w301, "Scale.Increment"=w299) -> ()  [unwired: 2 in, 2 out]
            n171 = property on="On/Off" class="Bool (strict)"("Visible"=w304) -> ()  [unwired: 2 in, 2 out]
            n172 = property on="Test Slider" class="Slide (strict)"("Visible"=w304) -> ()  [unwired: 2 in, 2 out]
            n173 = property on="Test Ring" class="Ring (strict)"("Visible"=w304) -> ()  [unwired: 2 in, 2 out]
            n174 = property on="Rev/Fwd" class="Clust (strict)"("Visible"=w304) -> ()  [unwired: 2 in, 2 out]
          }
          frame "Servo" {
            w320 = FALSE ("Visible")
            n175 = call <vilib>:"NT Read Number.vi"("Name"=w322) -> ("Numeric"=w321:dbl)  [unwired: 9 in, 1 out]
            n176 = property on="Test Slider" class="Slide (strict)"("Visible"=TRUE, "Scale.Maximum"=170.0 ("Scale.Range:Maximum")) -> ()  [unwired: 2 in, 2 out]
            n177 = local write "Test Slider"(w321) -> ()
            n178 = property on="Motor" class="Clust (strict)"("Visible"=w320) -> ()  [unwired: 2 in, 2 out]
            n179 = property on="Rev/Fwd" class="Clust (strict)"("Visible"=w320) -> ()  [unwired: 2 in, 2 out]
            n180 = property on="On/Off" class="Bool (strict)"("Visible"=w320) -> ()  [unwired: 2 in, 2 out]
            n181 = property on="Test Ring" class="Ring (strict)"("Visible"=w320) -> ()  [unwired: 2 in, 2 out]
          }
          frame "Relay", "Solenoid" {
            w323 = FALSE ("Visible")
            n182 = property on="Motor" class="Clust (strict)"("Visible"=w323) -> ()  [unwired: 2 in, 2 out]
            n183 = property on="Test Slider" class="Slide (strict)"("Visible"=w323) -> ()  [unwired: 2 in, 2 out]
            n184 = Search and Replace String(input string=w324, search string="/Value  **", replace string="/Direction") -> (result string=w330:string)  [unwired: 5 in, 3 out]
            n185 = property on="Test Ring" class="Ring (strict)"("Visible"=w323) -> ()  [unwired: 2 in, 2 out]
            n186 = call <vilib>:"NT Read String.vi"("Name"=w330) -> ("String"=w328:string)  [unwired: 9 in, 1 out]
            n187 = Equal?(x="Both directions", y=w328) -> (x = y?=w326:bool)
            n188 = Not(x=w326) -> (.not. x?=w327:bool)
            n189 = property on="Rev/Fwd" class="Clust (strict)"("Visible"=w326) -> ()  [unwired: 2 in, 2 out]
            n190 = property on="On/Off" class="Bool (strict)"("Visible"=w327, "Caption.Text"=w325) -> ()  [unwired: 2 in, 2 out]
          }
          frame "Compressor", "Digital Out" {
            w333 = FALSE ("Visible")
            # "Get direction and finish"
            n191 = property on="Motor" class="Clust (strict)"("Visible"=w333) -> ()  [unwired: 2 in, 2 out]
            n192 = property on="Test Slider" class="Slide (strict)"("Visible"=w333) -> ()  [unwired: 2 in, 2 out]
            n193 = property on="Test Ring" class="Ring (strict)"("Visible"=w333) -> ()  [unwired: 2 in, 2 out]
            n194 = property on="On/Off" class="Bool (strict)"("Visible"=TRUE, "Caption.Text"=w334) -> ()  [unwired: 2 in, 2 out]
            n195 = property on="Rev/Fwd" class="Clust (strict)"("Visible"=FALSE) -> ()  [unwired: 2 in, 2 out]
          }
          frame "Camera" {
            n196 = call <vilib>:"Get Last Path Segment.vi"("String in"=w341) -> ("String out"=w342:string)  [unwired: 10 in]
            n197 = property on="On/Off" class="Bool (strict)"("Visible"=FALSE) -> ()  [unwired: 2 in, 2 out]
            n198 = property on="Motor" class="Clust (strict)"("Visible"=FALSE) -> ()  [unwired: 2 in, 2 out]
            n199 = property on="Rev/Fwd" class="Clust (strict)"("Visible"=FALSE) -> ()  [unwired: 2 in, 2 out]
            n200 = case shown="\"White Balance  **\"" w342 {
              tunnel: w341 -> [w348 w357 w366 w375 w384 _ w390]
              tunnel: w340 -> [w346 w354 w363 w372 w381 _ _]
              frame "Size  **" {
                n201 = Index Array(array=w346) -> (element=w345:cluster{string[]})  [unwired: 1 in]
                n202 = call <vilib>:"NT Read String.vi"("Name"=w348) -> ("String"=w347:string)  [unwired: 9 in, 1 out]
                n203 = Unbundle(w345) -> (w343:string[])
                n204 = Match First String(2:w343, 3:w347) -> (0:w344:i32)  [unwired: 1 out]
                n205 = property on="Test Ring" class="Ring (strict)"("Value"=w344, "Strings []"=w343) -> ()  [unwired: 2 in, 2 out]
                n206 = property on="Test Ring" class="Ring (strict)"("Visible"=TRUE) -> ()  [unwired: 2 in, 2 out]
                n207 = property on="Test Slider" class="Slide (strict)"("Visible"=FALSE) -> ()  [unwired: 2 in, 2 out]
              }
              frame "White Balance  **" {
                n208 = Index Array(array=w354, index=1) -> (element=w355:cluster{string[]})
                n209 = call <vilib>:"NT Read String.vi"("Name"=w357) -> ("String"=w356:string)  [unwired: 9 in, 1 out]
                n210 = Unbundle(w355) -> (w352:string[])
                n211 = Match First String(2:w352, 3:w356) -> (0:w351:i32)  [unwired: 1 out]
                n212 = property on="Test Ring" class="Ring (strict)"("Value"=w351, "Strings []"=w352) -> ()  [unwired: 2 in, 2 out]
                n213 = property on="Test Ring" class="Ring (strict)"("Visible"=TRUE) -> ()  [unwired: 2 in, 2 out]
                n214 = property on="Test Slider" class="Slide (strict)"("Visible"=FALSE) -> ()  [unwired: 2 in, 2 out]
              }
              frame "Exposure  **" {
                n215 = Index Array(array=w363, index=2) -> (element=w364:cluster{string[]})
                n216 = call <vilib>:"NT Read String.vi"("Name"=w366) -> ("String"=w365:string)  [unwired: 9 in, 1 out]
                n217 = Unbundle(w364) -> (w360:string[])
                n218 = Match First String(2:w360, 3:w365) -> (0:w361:i32)  [unwired: 1 out]
                n219 = property on="Test Ring" class="Ring (strict)"("Value"=w361, "Strings []"=w360) -> ()  [unwired: 2 in, 2 out]
                n220 = property on="Test Ring" class="Ring (strict)"("Visible"=TRUE) -> ()  [unwired: 2 in, 2 out]
                n221 = property on="Test Slider" class="Slide (strict)"("Visible"=FALSE) -> ()  [unwired: 2 in, 2 out]
              }
              frame "Exposure Priority  **" {
                n222 = Index Array(array=w372, index=3) -> (element=w373:cluster{string[]})
                n223 = call <vilib>:"NT Read String.vi"("Name"=w375) -> ("String"=w374:string)  [unwired: 9 in, 1 out]
                n224 = Unbundle(w373) -> (w369:string[])
                n225 = Match First String(2:w369, 3:w374) -> (0:w370:i32)  [unwired: 1 out]
                n226 = property on="Test Ring" class="Ring (strict)"("Value"=w370, "Strings []"=w369) -> ()  [unwired: 2 in, 2 out]
                n227 = property on="Test Ring" class="Ring (strict)"("Visible"=TRUE) -> ()  [unwired: 2 in, 2 out]
                n228 = property on="Test Slider" class="Slide (strict)"("Visible"=FALSE) -> ()  [unwired: 2 in, 2 out]
              }
              frame "Color Enable  **" {
                n229 = Index Array(array=w381, index=4) -> (element=w382:cluster{string[]})
                n230 = call <vilib>:"NT Read String.vi"("Name"=w384) -> ("String"=w383:string)  [unwired: 9 in, 1 out]
                n231 = Unbundle(w382) -> (w378:string[])
                n232 = Match First String(2:w378, 3:w383) -> (0:w379:i32)  [unwired: 1 out]
                n233 = property on="Test Ring" class="Ring (strict)"("Value"=w379, "Strings []"=w378) -> ()  [unwired: 2 in, 2 out]
                n234 = property on="Test Ring" class="Ring (strict)"("Visible"=TRUE) -> ()  [unwired: 2 in, 2 out]
                n235 = property on="Test Slider" class="Slide (strict)"("Visible"=FALSE) -> ()  [unwired: 2 in, 2 out]
              }
              frame Default {
                n236 = property on="Test Ring" class="Ring (strict)"("Visible"=FALSE) -> ()  [unwired: 2 in, 2 out]
                n237 = property on="Test Slider" class="Slide (strict)"("Visible"=FALSE) -> ()  [unwired: 2 in, 2 out]
              }
              frame "Brightness  **", "Color Level  **", "Compression  **", "FPS  **", "Sharpness  **" {
                n238 = call <vilib>:"NT Read Number.vi"("Name"=w390) -> ("Numeric"=w389:dbl)  [unwired: 9 in, 1 out]
                n239 = local write "Test Slider"(w389) -> ()
                n240 = property on="Test Slider" class="Slide (strict)"("Visible"=TRUE, "Scale.Maximum"=100.0 ("Scale.Range:Maximum")) -> ()  [unwired: 2 in, 2 out]
                n241 = property on="Test Ring" class="Ring (strict)"("Visible"=FALSE) -> ()  [unwired: 2 in, 2 out]
              }
            }
          }
        }
        n242 = property on="Progress" class="Clust (strict)"("Visible"=FALSE) -> ()  [unwired: 2 in, 2 out]
      }
      event "Test Name": Mouse Enter {
        # "Populate the ring with the list of tests"
        n243 = event-data() -> ()  [unwired: 1 in, 1 out]
        n244 = call <vilib>:"NT Read String Array.vi"("Name"="/TestMode/TestList") -> ("String Array"=w398:string[])  [unwired: 9 in, 1 out]
        n245 = Build Array (concatenate)("Select the test to run...", w398) -> (w397:string[])
        n246 = property on="Test Name" class="Ring (strict)"("Strings []"=w397) -> ()  [unwired: 2 in, 2 out]
      }
      event "Test Name": Value Change {
        w400 = FALSE ("Visible")
        # "Tell the robot the test name to run"
        n247 = event-data() -> ("NewVal"=w404:u16)  [unwired: 1 in]
        n248 = property on="Test Name" class="Ring (strict)"() -> ("Strings []"=w405:string[])  [unwired: 2 in, 2 out]
        n249 = local write "Progress"(T6 {"Test Progress"=0, "Test Progress Text"=""} ("Progress")) -> ()
        n250 = Index Array(array=w405, index=w404) -> (element=w403:string)
        n251 = call <vilib>:"NT Write String.vi"("String"=w403, "Name"="/TestMode/TestName") -> ()  [unwired: 9 in, 1 out]
        n252 = property on="Progress" class="Clust (strict)"("Visible"=TRUE) -> ()  [unwired: 2 in, 2 out]
        n253 = property on="Motor" class="Clust (strict)"("Visible"=w400) -> ()  [unwired: 2 in, 2 out]
        n254 = property on="Test Slider" class="Slide (strict)"("Visible"=w400) -> ()  [unwired: 2 in, 2 out]
        n255 = property on="On/Off" class="Bool (strict)"("Visible"=w400) -> ()  [unwired: 2 in, 2 out]
        n256 = property on="Rev/Fwd" class="Clust (strict)"("Visible"=w400) -> ()  [unwired: 2 in, 2 out]
        n257 = property on="Test Ring" class="Ring (strict)"("Visible"=w400) -> ()  [unwired: 2 in, 2 out]
      }
      event "Select Auto": Mouse Enter {
        # "Populate the combo box with the list of autonomous options"
        n258 = event-data() -> ()  [unwired: 1 in, 1 out]
        n259 = call <vilib>:"NT Read String Array.vi"("Name"="Auto List") -> ("String Array"=w407:string[])  [unwired: 9 in, 1 out]
        n260 = property on="Select Auto" class="CmbBox"("Strings[]"=w407) -> ()  [unwired: 2 in, 2 out]
      }
      event "Select Auto": Value Change {
        # "User modified the Auto Selection. Write to NT variable so robot knows."
        n261 = event-data() -> ("NewVal"=w410:string)  [unwired: 1 in]
        n262 = call <vilib>:"NT Write String.vi"("String"=w410, "Name"="Auto Selector") -> ()  [unwired: 9 in, 1 out]
      }
      event "Command Selection": Value Change {
        # "Get the params and show in table"
        n263 = event-data() -> ("NewVal"=w416:i32)  [unwired: 1 in]
        n264 = property on="Command Selection" class="MCListbox (strict)"() -> ("ItemNames"=w414:string[][])  [unwired: 2 in, 2 out]
        n265 = call <vilib>:"WPI_DashboardUpdate Command Params.vi"("NewVal"=w416, "Commands"=w414, "Param Tbl"=w415) -> ()  [unwired: 8 in, 1 out]
      }
      event "Execute Command": Value Change {
        # "Started one, Unique ID holds\nresponse"
        n266 = event-data() -> ()  [unwired: 1 in, 1 out]
        n267 = property on="Command Selection" class="MCListbox (strict)"() -> ("ItemNames"=w427:string[][])  [unwired: 2 in, 2 out]
        n268 = Index Array(array=w427, index (row)="Command Selection", index (col)=0) -> (element=w425:string)
        n269 = call <vilib>:"Invoke Commands.vi"("Command Params"="Command Params", "Function Name"=w425) -> ("Params"=w421:u8, "Started"=w420:bool)  [unwired: 7 in, 1 out]
        n270 = Array Subset(array="Command Params", length (row)=w421) -> (w422:string[][])  [unwired: 3 in]
        n271 = Select(t="Executing" ("Cmd Status"), s=w420, f="" ("Cmd Status")) -> (s? t:f=→"Cmd Status":string)
      }
      event "Command Selection": Double Click {
        n272 = event-data() -> ("Row"=w435:i32)  [unwired: 1 in]
        n273 = property on="Command Selection" class="MCListbox (strict)"() -> ("ItemNames"=w438:string[][])  [unwired: 2 in, 2 out]
        n274 = local read "Command Params"() -> (w434:string[][])
        n275 = Index Array(array=w438, index (row)=w435, index (col)=0) -> (element=w436:string)
        n276 = call <vilib>:"Invoke Commands.vi"("Command Params"=w434, "Function Name"=w436) -> ("Params"=w433:u8, "Started"=w428:bool)  [unwired: 7 in, 1 out]
        n277 = Array Subset(array=w434, length (row)=w433) -> (w432:string[][])  [unwired: 3 in]
        n278 = Select(t="Executing" ("Cmd Status"), s=w428, f="" ("Cmd Status")) -> (s? t:f=w429:string)
        n279 = local write "Cmd Status"(w429) -> ()
      }
      event "CheckList": Double Click {
        # "Shift clears all"
        # "Update symbols on the listbox"
        n280 = event-data() -> ("PlatMods.Shift"=w440:bool, "Row"=w442:i32)  [unwired: 1 in]
        n281 = case shown="True" w440 {
          tunnel: w442 -> [w446 _]
          tunnel: 1 -> [w445 _]
          frame False {
            n282 = property on="CheckList" class="LstBox (strict)"() -> ("Item Symbols"=w444:i32[])  [unwired: 2 in, 2 out]
            n283 = Replace Array Subset(array=w444, new element=w445, index=w446) -> (w443:i32[])
            n284 = property on="CheckList" class="LstBox (strict)"("Item Symbols"=w443) -> ()  [unwired: 2 in, 2 out]
          }
          frame True {
            w447 = 0 ("Top Row")
            n285 = property on="CheckList" class="LstBox (strict)"() -> ("Number of Rows"=w449:u32)  [unwired: 2 in, 2 out]
            n286 = Initialize Array(0, w449) -> (w448:i32[])
            n287 = property on="CheckList" class="LstBox (strict)"("Top Row"=w447, "Value"=w447, "Item Symbols"=w448) -> ()  [unwired: 2 in, 2 out]
          }
        }
      }
      event "CheckList": Key Down {
        # "Update symbols on the listbox\nLeft and right keys check and uncheck"
        n288 = event-data() -> ("VKey"=w453:T21)  [unwired: 1 in]
        n289 = case shown="\"Left\", \"Right\"" w453 {
          selector: w453 -> [w458 _]
          tunnel: eventvkey."Left" ("VKey") -> [w456 _]
          frame "Left", "Right" {
            n290 = Equal?(x=w456, y=w458) -> (x = y?=w457:bool)
            n291 = Select(t=0, s=w457, f=1) -> (s? t:f=w459:i32)
            n292 = property on="CheckList" class="LstBox (strict)"() -> ("Item Symbols"=w462:i32[])  [unwired: 2 in, 2 out]
            n293 = Replace Array Subset(array=w462, new element=w459, index="CheckList") -> (w461:i32[])
            n294 = property on="CheckList" class="LstBox (strict)"("Item Symbols"=w461) -> ()  [unwired: 2 in, 2 out]
          }
          frame Default {
          }
        }
      }
      event "Motor.Enable": Value Change {
        # "When the test mode otor enable helper is set, update that\ntree row item's value"
        n295 = event-data() -> ("NewVal"=w468:bool)  [unwired: 1 in]
        n296 = Unbundle("Motor") -> ("Value"=w467:dbl)  [unwired: 1 out]
        n297 = Select(t=w467, s=w468, f=0.0) -> (s? t:f=w465:dbl)
        n298 = call <vilib>:"NT Write Number.vi"("Numeric"=w465, "Name"=w464) -> ()  [unwired: 9 in, 1 out]
      }
      event "Test Slider": Value Change {
        # "When the test mode slider helper is set, update that\ntree row item's value"
        n299 = event-data() -> ("NewVal"=w471:dbl)  [unwired: 1 in]
        n300 = call <vilib>:"NT Write Number.vi"("Numeric"=w471, "Name"=w472) -> ()  [unwired: 9 in, 1 out]
      }
      event "On/Off": Value Change {
        # "When the test mode on/off helper value is set, update that\ntree row item's value"
        n301 = event-data() -> ("NewVal"=w476:bool)  [unwired: 1 in]
        n302 = Boolean To (0,1)(Boolean=w476) -> (0, 1=w475:i16)
        n303 = call <vilib>:"NT Write Number.vi"("Numeric"=w475, "Name"=w474) -> ()  [unwired: 9 in, 1 out]
      }
      event "Rev/Fwd": Value Change {
        # "When the test mode helper value for relays is set, update that\ntree row item's value"
        n304 = event-data() -> ("NewVal.Forward"=w484:bool, "NewVal.Reverse"=w483:bool)  [unwired: 1 in]
        n305 = Boolean To (0,1)(Boolean=w484) -> (0, 1=w480:i16)
        n306 = Boolean To (0,1)(Boolean=w483) -> (0, 1=w482:i16)
        n307 = Negate(x=w482) -> (-x=w481:i16)
        n308 = Add(x=w480, y=w481) -> (x+y=w479:i16)
        n309 = call <vilib>:"NT Write Number.vi"("Numeric"=w479, "Name"=w478) -> ()  [unwired: 9 in, 1 out]
      }
      event "Test Ring": Value Change {
        # "When a test mode helper value is selected from the ring,\nset the tree item's variable to the string value"
        n310 = event-data() -> ("NewVal"=w488:u16)  [unwired: 1 in]
        n311 = property on="Test Ring" class="Ring (strict)"() -> ("Strings []"=w489:string[])  [unwired: 2 in, 2 out]
        n312 = Index Array(array=w489, index=w488) -> (element=w487:string)
        n313 = call <vilib>:"NT Write String.vi"("String"=w487, "Name"=w486) -> ()  [unwired: 9 in, 1 out]
      }
      event "Rec Mode": Value Change {
        # "Update globals for recording mode and path to read log from.\nClear when logging and let NetworkTables set path for vision to\nuse."
        n314 = event-data() -> ("NewVal"=w500:enum32{"Stop", "Record", "Playback"})  [unwired: 1 in]
        n315 = global write "WPI_DashboardLogging Global.vi" "Logging Filename"(path "") -> ()
        n316 = global write "WPI_DashboardLogging Global.vi" "Recording"(w500) -> ()
        n317 = case shown="\"Playback\"" w500 {
          tunnel: w499 -> [_ w502 w511]
          tunnel: [_ _ w510] -> w497
          tunnel: [_ _ w509] -> _
          tunnel: w495 -> [_ _ w507]
          tunnel: cluster{i32, i32} {-250, 170} -> [_ _ w506]
          tunnel: [_ _ T22 {"Image Size"=TRUE, "Image Type"=TRUE, "Pixel Value"=TRUE, "ROI Information"=TRUE, "Zoom Factor"=FALSE} ("Image Information Shown:All Elements")] -> w493
          tunnel: [_ _ TRUE ("Zoom Factor")] -> w492
          tunnel: w491 -> [_ _ w503]
          frame Default {
          }
          frame "Stop", "Record" {
            # "Place Window too"
            n318 = invoke class="VI" method="FP.Close"(reference=w502) -> (reference out=w501:refnum<vi>)  [unwired: 2 in, 2 out]
            n319 = invoke class="VI" method="Abort VI"(reference=w501) -> ()  [unwired: 2 in, 3 out]
          }
          frame "Playback" {
            n320 = call "Open Playback Panel.vi"("Offset"=w506, "DB VI Ref"=w507, "Playback in"=w511) -> ("Playback out"=w508:refnum<vi>)  [unwired: 8 in]
            n321 = register-events(w508, w503) -> (reference out=w510:refnum<event-registration>, error out=w509:errorcluster)  [unwired: 2 in]
          }
        }
        n322 = property on="Camera Image" class="ImageControl"("Image Information Shown"=w493, "Image Information Visible"=w492) -> ()  [unwired: 2 in, 2 out]
        n323 = call <vilib>:"WPI_DashboardNT Log FieldName Cache.vi"("Operation"=enum16{"Lookup/Add", "Index", "Clear"}."Clear") -> ()  [unwired: 8 in, 3 out]
      }
      event Panel Close {
        w513 = enum32{"Stop", "Record", "Playback"}."Stop" ("Rec Mode")
        # "Playback window has been closed, abort"
        n324 = event-data() -> ()  [unwired: 1 in, 4 out]
        n325 = local write "Rec Mode"(w513) -> ()
        n326 = global write "WPI_DashboardLogging Global.vi" "Recording"(w513) -> ()
      }
      event Panel Close {
        # "Abort playback window and ourself"
        n327 = event-data() -> ()  [unwired: 1 in, 4 out]
        n328 = invoke class="VI" method="FP.Close"(reference=w517) -> (reference out=w516:refnum<vi>)  [unwired: 2 in, 2 out]
        n329 = invoke class="VI" method="Abort VI"(reference=w516) -> (error out=w515:errorcluster)  [unwired: 2 in, 2 out]
        n330 = invoke class="VI" method="Abort VI"(error in=w515) -> ()  [unwired: 2 in, 3 out]
      }
      event User Event {
        n331 = event-data() -> ("IDs"=w524:cluster{"RPC field ID":u16, "Unique ID":u16}, "String"=w523:string)  [unwired: 1 in]
        n332 = Bundle("IDs"=w524, "String"=w523) -> (w522:T8)  [unwired: 1 in]
        n333 = call <vilib>:"Retrieve RPC Response.vi"("RPC Response"=w522) -> ("Output"=w520:string[][])  [unwired: 10 in]
        n334 = Build Array (concatenate)(w518, w520) -> (w519:string[][])
        n335 = local write "Command Params"(w519) -> ()
        n336 = local write "Cmd Status"("" ("Cmd Status")) -> ()
      }
      event "Tree": Double Click {
        n337 = event-data() -> ("PlatMods"=w528:T25, "Tag"=w527:string)  [unwired: 1 in]
        n338 = Unbundle(w528) -> ("Shift"=w526:bool)  [unwired: 4 out]
        n339 = Not(x=w526) -> (.not. x?=w525:bool)
        n340 = call <vilib>:"NT Update Persistence.vi"("Persistence"=w525, "Name"=w527) -> ()  [unwired: 9 in, 1 out]
      }
    }
  }
  n341 = while {
    tunnel: w64 -> [w531]
    i -> [w534]
    stop <- FALSE stop-if-true
    n342 = Wait (ms)(milliseconds to wait=u32 100) -> ()  [unwired: 1 out]
    n343 = case shown="\"Playback\"" "Rec Mode" {
      tunnel: w534 -> [_ _ w549]
      tunnel: [u32 2829099 ("Base Color") u32 11141120 ("Target Color") w538] -> w530
      frame "Stop", Default {
        # "Reset the color, extra updates don't cost much"
      }
      frame "Record" {
      }
      frame "Playback" {
        # "Playback"
        n344 = Quotient & Remainder(x=w549, y=u32 50 ("milliseconds to wait")) -> (x-y*floor(x/y)=w545:u32)  [unwired: 1 out]
        n345 = Divide(x=w545, y=u32 50 ("milliseconds to wait")) -> (x/y=w542:dbl)
        n346 = Multiply(x=6.283185307179586, y=w542) -> (x*y=w547:dbl)
        n347 = Sine(x=w547) -> (sin(x)=w546:dbl)
        n348 = Absolute Value(x=w546) -> (abs(x)=w539:dbl)
        n349 = call "Interpolate RGB Color.vi"("Proportion"=w539, "Target Color"=u32 30976, "Base Color"=u32 2829099) -> ("Result Color"=w538:u32)  [unwired: 8 in]
      }
    }
    n350 = property class="Pane"(reference=w531, "PaneColor"=w530) -> ()  [unwired: 1 in, 2 out]
  }
  n351 = local write "Dashboard Tab"(T9."Drive" ("Dashboard Tab")) -> ()
  n352 = property on="On/Off" class="Bool (strict)"("Visible"=w33) -> ()  [unwired: 2 in, 2 out]
  n353 = property on="Motor" class="Clust (strict)"("Visible"=w33) -> ()  [unwired: 2 in, 2 out]
  n354 = property on="Progress" class="Clust (strict)"("Visible"=w33) -> ()  [unwired: 2 in, 2 out]
  n355 = property on="Test Ring" class="Ring (strict)"("Visible"=w33) -> ()  [unwired: 2 in, 2 out]
  n356 = property on="Rev/Fwd" class="Clust (strict)"("Visible"=w33) -> ()  [unwired: 2 in, 2 out]
  n357 = local write "Command Selection"(u16 0 ("milliseconds to wait")) -> ()
  n358 = local write "Command Params"(string[][] [] ("Command Params")) -> ()
  n359 = global write "WPI_DashboardLogging Global.vi" "Recording"(w58) -> ()
  n360 = local write "Rec Mode"(w58) -> ()
  n361 = while {
    tunnel: u16 1741 ("timeout ms (25000)") -> [w551]
    stop <- FALSE stop-if-true
    n362 = TCP Create Listener(10:w551) -> (0:w550:errorcluster, 3:w552:refnum<k5>)  [unwired: 4 in, 1 out]
    n363 = case shown="No Error" w550 {
      selector: w550 -> [w554 _]
      tunnel: w552 -> [w555 _]
      frame No Error {
        n364 = while {
          tunnel: w555 -> [w558]
          tunnel: w554 -> [w557]
          stop <- FALSE stop-if-true
          n365 = TCP Wait On Listener(8:w557, 11:w558) -> (0:w559:errorcluster, 4:w560:refnum<k5>)  [unwired: 2 in, 3 out]
          n366 = local write "TCP"(w560) -> ()
          n367 = case shown="No Error" w559 {
            frame No Error {
            }
            frame Error {
              n368 = Wait (ms)(milliseconds to wait=u32 1000) -> ()  [unwired: 1 out]
            }
          }
        }
      }
      frame Error {
        n369 = Wait (ms)(milliseconds to wait=u32 1000) -> ()  [unwired: 1 out]
      }
    }
  }
  n370 = call <vilib>:"NT Write String.vi"("String"="Select Auto", "Name"="Auto Selector") -> ()  [unwired: 9 in, 1 out]
